vi "Get Travel Speed.vi"(8 "error in (no error)":errorcluster, 11 "ESM303 in":refnum<class "ESM303.lvclass">) -> (0 "error out":errorcluster, 1 "Speed Units":T1, 2 "Speed":dbl format="%.3f", 3 "ESM303 out":refnum<class "ESM303.lvclass">)   [LabVIEW 2018, in "ESM303.lvlib" / "ESM303.lvclass"]
uses:
  ESM303.lvclass
  builds/Force Test Stand/Force Test Stand/Force Test Stand.lvlibp/Custom Controls/Speed Units.ctl
  builds/Force Test Stand/Force Test Stand/Force Test Stand.lvlibp/Force Test Stand.lvclass
  C:/Projects/LabVIEW/In-Progress/Jose Rivero-Diaz/builds/Force Test Stand/Force Test Stand/Force Test Stand.lvlibp/Force Test Stand.lvclass
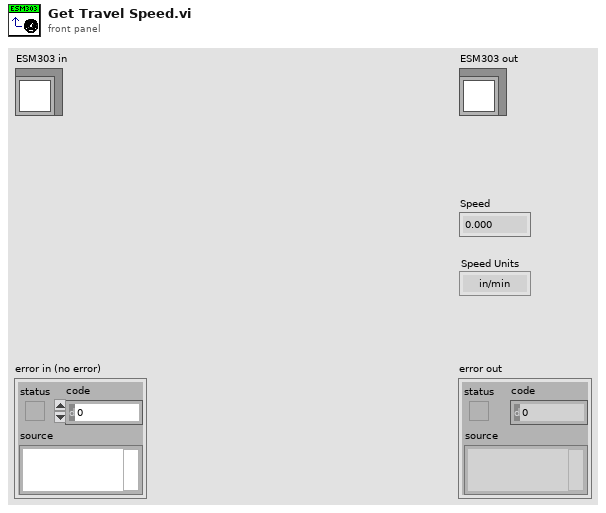
[diagram p1: front panel]
types:
  T1 = typedef "Force Test Stand.lvlibp/Force Test Stand.lvclass/Speed Units.ctl" = enum16{"in/min", "mm/min"}
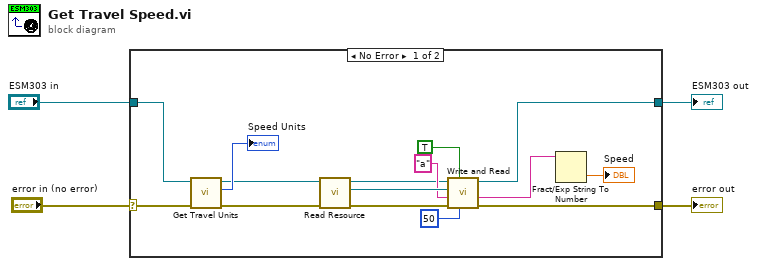
[diagram p0: block diagram]
diagram:
  n1 = case shown="No Error" "error in (no error)" {
    selector: "error in (no error)" -> [w9 w21]
    tunnel: [w18 w21] -> w3
    tunnel: [w11 w20] -> w2
    tunnel: "ESM303 in" -> [w10 w20]
    frame No Error {
      n2 = call-dynamic "Get Travel Units.vi"("error in (no error)"=w9, "ESM303 in"=w10) -> ("error out"=w7:errorcluster, "Travel Units"=→"Speed Units":T1, "ESM303 out"=w8:refnum<class "ESM303.lvclass">)  [unwired: 7 in]
      n3 = call "Read Resource.vi"("error in (no error)"=w7, "Force Test Stand in"=w8) -> ("error out"=w5:errorcluster, "Resource"=w17:refnum<visa-resource-name>, "Force Test Stand out"=w6:refnum<class "ESM303.lvclass">)  [unwired: 7 in]
      n4 = call "Write and Read.vi"("Delay Before Read (ms)"=50, "Write & Read"=TRUE, "error in (no error)"=w5, "Command"="a", "VISA Refnum in"=w17, "ESM303 in"=w6) -> ("error out"=w18:errorcluster, "Response"=w13:string, "ESM303 out"=w11:refnum<class "ESM303.lvclass">)  [unwired: 3 in]
      n5 = Fract/Exp String To Number(string=w13) -> (number=→"Speed":dbl)  [unwired: 3 in, 1 out]
    }
    frame Error {
    }
  }
  "error out" <- w3
  "ESM303 out" <- w2
